vi "Configure Library on Disk for Build.vi"(9 "enable debugging? (F)":bool, 10 "save VIs? (T)":bool=TRUE, 11 "library path":path) -> (0 "error out":errorcluster)   [LabVIEW 2017, in "Build Automation.lvlib"]
uses:
  Build Automation.lvlib
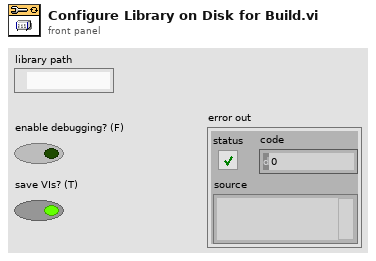
[diagram p1: front panel]
types:
  T1 = enum16{"Share clones between instances", "Preallocate clone for each instance"}
  T2 = cluster{"Status Message":refnum<data-value>, "Progress":refnum<data-value>, "Stop":refnum<data-value>}
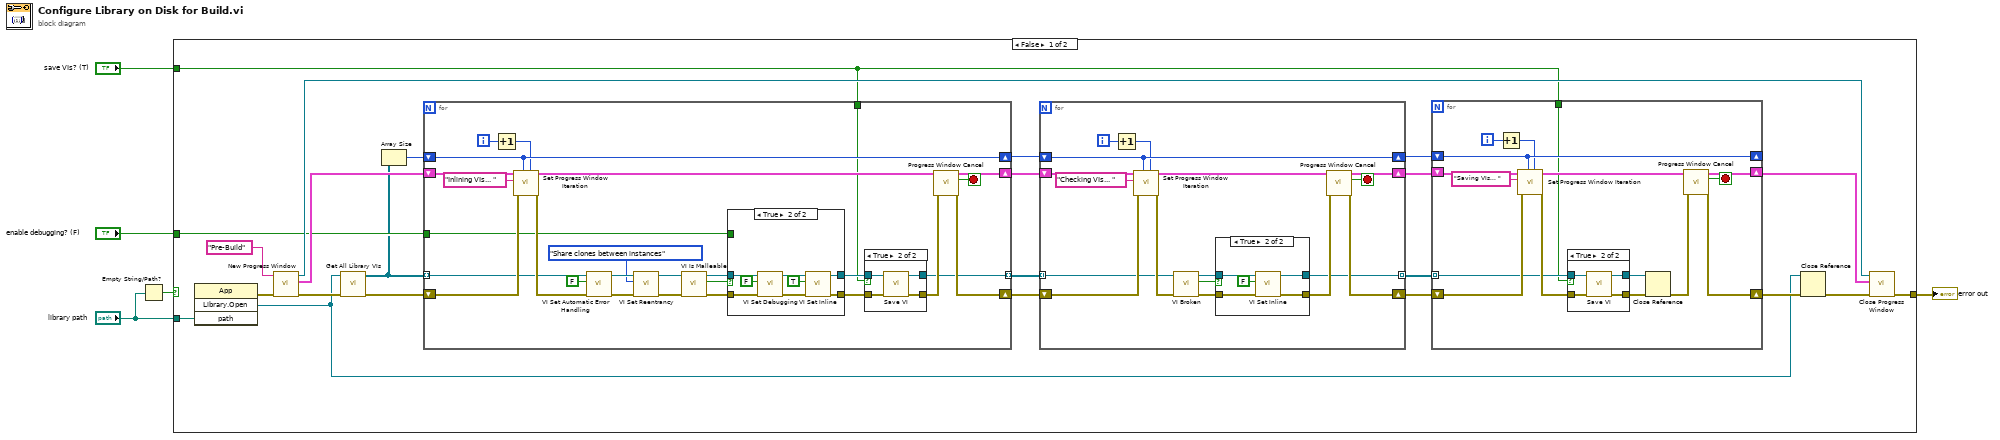
[diagram p0: block diagram]
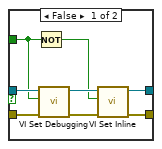
[diagram p3: hidden frame]
diagram:
  n1 = Empty String/Path?(string/path="library path") -> (empty?=w3:bool)
  n2 = case shown="False" w3 {
    tunnel: [w25 _] -> w5
    tunnel: "enable debugging? (F)" -> [w24 _]
    tunnel: "save VIs? (T)" -> [w6 _]
    tunnel: "library path" -> [w7 _]
    frame False {
      n3 = invoke class="App" method="Library.Open"("path"=w7) -> (error out=w8:errorcluster, "Open Library"=w9:refnum<vi>)  [unwired: 3 in, 2 out]
      n4 = call "New Progress Window.vi"("error in (no error)"=w8, "WindowTitle"="Pre-Build") -> ("error out"=w27:errorcluster, "DVRs"=w26:T2, "VI refnum"=w28:refnum<vi>)  [unwired: 7 in]
      n5 = call "Get All Library VIs.vi"("error in (no error)"=w27, "library ref"=w9) -> ("error out"=w29:errorcluster, "vi refs"=w22:refnum<vi>[])  [unwired: 8 in]
      n6 = Array Size(array=w22) -> (size(s)=w23:i32)
      n7 = for {
        tunnel: w22 -> [w39] mode=indexing
        shift-right: [w54] -> w20
        shift-left: w26 -> [w44]
        shift-right: [w40] -> w18
        shift-left: w29 -> [w42]
        tunnel: w24 -> [w38]
        tunnel: [w31] -> w19 mode=indexing
        shift-right: [w37] -> w21
        shift-left: w23 -> [w37]
        tunnel: w6 -> [w30]
        i -> [w56]
        stop <- w55 stop-if-true
        n8 = Increment(x=w56) -> (x+1=w36:i32)
        n9 = call "Set Progress Window Iteration.vi"("current iteration"=w36, "total iterations"=w37, "error in (no error)"=w42, "Status Message"="Inlining VIs... ", "DVRs in"=w44) -> ("error out"=w41:errorcluster, "DVRs out"=w43:T2)  [unwired: 5 in]
        n10 = call "VI Set Automatic Error Handling.vi"("error in (no error)"=w41, "Automatic Error Handling"=FALSE, "vi ref in"=w39) -> ("error out"=w51:errorcluster, "vi ref out"=w52:refnum<vi>)  [unwired: 7 in]
        n11 = call "VI Set Reentrancy.vi"("error in (no error)"=w51, "Reentrancy Type"=T1."Share clones between instances", "vi ref in"=w52) -> ("error out"=w48:errorcluster, "vi ref out"=w49:refnum<vi>)  [unwired: 7 in]
        n12 = call "VI Is Malleable.vi"("error in (no error)"=w48, "vi ref in"=w49) -> ("error out"=w47:errorcluster, "malleable VI?"=w45:bool, "vi ref out"=w46:refnum<vi>)  [unwired: 7 in]
        n13 = case shown="True" w45 {
          tunnel: [w68 w76] -> w33
          tunnel: [w67 w75] -> w34
          tunnel: w47 -> [w64 w73]
          tunnel: w46 -> [w65 w74]
          tunnel: w38 -> [w63 _]
          frame False {
            n14 = Not(x=w63) -> (.not. x?=w66:bool)
            n15 = call "VI Set Debugging.vi"("error in (no error)"=w64, "Allow Debugging"=w63, "vi ref in"=w65) -> ("error out"=w69:errorcluster, "vi ref out"=w70:refnum<vi>)  [unwired: 7 in]
            n16 = call "VI Set Inline.vi"("error in (no error)"=w69, "Inline VI"=w66, "vi ref in"=w70) -> ("error out"=w67:errorcluster, "vi ref out"=w68:refnum<vi>)  [unwired: 7 in]
          }
          frame True {
            n17 = call "VI Set Debugging.vi"("error in (no error)"=w73, "Allow Debugging"=FALSE, "vi ref in"=w74) -> ("error out"=w77:errorcluster, "vi ref out"=w78:refnum<vi>)  [unwired: 7 in]
            n18 = call "VI Set Inline.vi"("error in (no error)"=w77, "Inline VI"=TRUE, "vi ref in"=w78) -> ("error out"=w75:errorcluster, "vi ref out"=w76:refnum<vi>)  [unwired: 7 in]
          }
        }
        n19 = case shown="True" w30 {
          tunnel: w34 -> [w57 w62]
          tunnel: [w58 w61] -> w31
          tunnel: [w57 w60] -> w32
          tunnel: w33 -> [w58 w59]
          frame False {
          }
          frame True {
            n20 = call "Save VI.vi"("error in (no error)"=w62, "vi ref in"=w59) -> ("error out"=w60:errorcluster, "vi ref out"=w61:refnum<vi>)  [unwired: 8 in]
          }
        }
        n21 = call "Progress Window Cancel.vi"("error in (no error)"=w32, "DVRs in"=w43) -> ("error out"=w40:errorcluster, "cancelled"=w55:bool, "DVRs out"=w54:T2)  [unwired: 7 in]
      }
      n22 = for {
        tunnel: w19 -> [w84] mode=indexing
        shift-right: [w93] -> w17
        shift-left: w20 -> [w92]
        shift-right: [w89] -> w15
        shift-left: w18 -> [w90]
        shift-right: [w88] -> w16
        shift-left: w21 -> [w88]
        tunnel: [w79] -> w14 mode=indexing
        i -> [w95]
        stop <- w94 stop-if-true
        n23 = Increment(x=w95) -> (x+1=w87:i32)
        n24 = call "Set Progress Window Iteration.vi"("current iteration"=w87, "total iterations"=w88, "error in (no error)"=w90, "Status Message"="Checking VIs... ", "DVRs in"=w92) -> ("error out"=w85:errorcluster, "DVRs out"=w91:T2)  [unwired: 5 in]
        n25 = call "VI Broken.vi"("error in (no error)"=w85, "vi ref in"=w84) -> ("error out"=w82:errorcluster, "broken?"=w81:bool, "vi ref out"=w83:refnum<vi>)  [unwired: 7 in]
        n26 = case shown="True" w81 {
          tunnel: [w97 w102] -> w79
          tunnel: [w96 w101] -> w80
          tunnel: w82 -> [w96 w100]
          tunnel: w83 -> [w97 w98]
          frame False {
          }
          frame True {
            n27 = call "VI Set Inline.vi"("error in (no error)"=w100, "Inline VI"=FALSE, "vi ref in"=w98) -> ("error out"=w101:errorcluster, "vi ref out"=w102:refnum<vi>)  [unwired: 7 in]
          }
        }
        n28 = call "Progress Window Cancel.vi"("error in (no error)"=w80, "DVRs in"=w91) -> ("error out"=w89:errorcluster, "cancelled"=w94:bool, "DVRs out"=w93:T2)  [unwired: 7 in]
      }
      n29 = for {
        tunnel: w14 -> [w104] mode=indexing
        shift-right: [w116] -> w13
        shift-left: w17 -> [w115]
        shift-right: [w112] -> w11
        shift-left: w15 -> [w113]
        shift-right: [w111] -> _
        shift-left: w16 -> [w111]
        tunnel: w6 -> [w103]
        i -> [w118]
        stop <- w117 stop-if-true
        n30 = Increment(x=w118) -> (x+1=w110:i32)
        n31 = call "Set Progress Window Iteration.vi"("current iteration"=w110, "total iterations"=w111, "error in (no error)"=w113, "Status Message"="Saving VIs... ", "DVRs in"=w115) -> ("error out"=w105:errorcluster, "DVRs out"=w114:T2)  [unwired: 5 in]
        n32 = case shown="True" w103 {
          tunnel: w105 -> [w119 w124]
          tunnel: [w120 w123] -> w108
          tunnel: [w119 w122] -> w107
          tunnel: w104 -> [w120 w121]
          frame False {
          }
          frame True {
            n33 = call "Save VI.vi"("error in (no error)"=w124, "vi ref in"=w121) -> ("error out"=w122:errorcluster, "vi ref out"=w123:refnum<vi>)  [unwired: 8 in]
          }
        }
        n34 = Close Reference(reference=w108, error in (no error)=w107) -> (error out=w106:errorcluster)
        n35 = call "Progress Window Cancel.vi"("error in (no error)"=w106, "DVRs in"=w114) -> ("error out"=w112:errorcluster, "cancelled"=w117:bool, "DVRs out"=w116:T2)  [unwired: 7 in]
      }
      n36 = Close Reference(reference=w9, error in (no error)=w11) -> (error out=w10:errorcluster)
      n37 = call "Close Progress Window.vi"("error in (no error)"=w10, "DVRs in"=w13, "VI refnum"=w28) -> ("error out"=w25:errorcluster)  [unwired: 8 in]
    }
    frame True {
    }
  }
  "error out" <- w5
